vi "SSC Digital Clock Generator Initiate.vi"(0 "Digital SSC in":T1[](array[typedef]), 11 "error in":errorcluster) -> (4 "Digital SSC out":T1[](array[typedef]), 15 "error out":errorcluster)   [LabVIEW 2019]
doc: "Initiates clock generation on the device(s) connected to the specified pin(s) and pin group(s)."
uses:
  SSC Digital.ctl
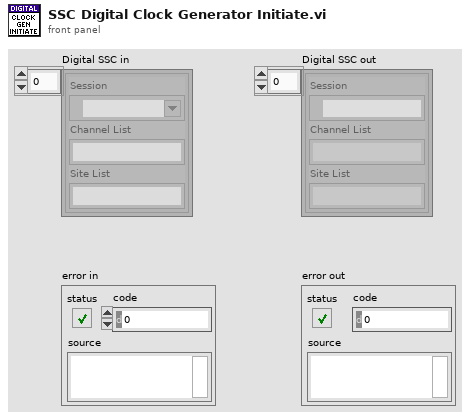
[diagram p1: front panel]
types:
  T1 = typedef "SSC Digital.ctl" = cluster{"Session":refnum<k15>, "Channel List":string, "Site List":string}
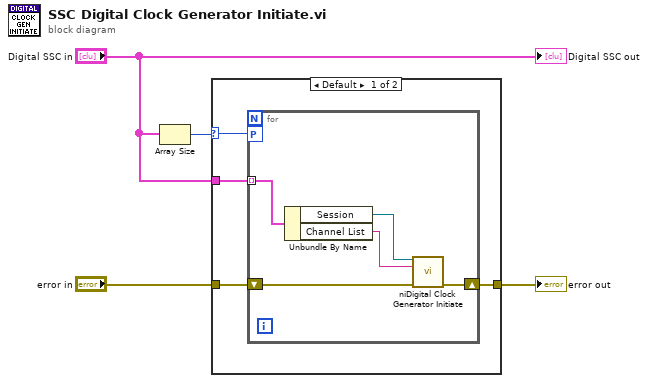
[diagram p0: block diagram]
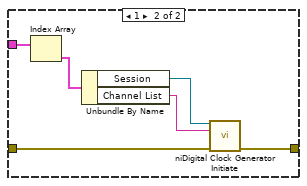
[diagram p2: hidden frame]
diagram:
  n1 = Array Size(array="Digital SSC in") -> (size(s)=w2:i32)
  n2 = case shown="Default" w2 {
    selector: w2 -> [w6 _]
    tunnel: "error in" -> [w8 w19]
    tunnel: [w7 w18] -> w3
    tunnel: "Digital SSC in" -> [w5 w17]
    frame Default {
      n3 = for {
        workers-P: w6 -> [_]
        tunnel: w5 -> [w12] mode=indexing
        shift-right: [w9] -> w7
        shift-left: w8 -> [w13]
        n4 = Unbundle By Name(w12) -> ("Session"=w11:refnum<k15>, "Channel List"=w10:string)
        n5 = call <instrlib>:"niDigital Clock Generator Initiate.vi"("instrument handle"=w11, "channel list"=w10, "error in"=w13) -> ("error out"=w9:errorcluster)  [unwired: 11 in, 1 out]
      }
    }
    frame 1 {
      n6 = Index Array(array=w17) -> (element=w14:T1)  [unwired: 1 in]
      n7 = Unbundle By Name(w14) -> ("Session"=w16:refnum<k15>, "Channel List"=w15:string)
      n8 = call <instrlib>:"niDigital Clock Generator Initiate.vi"("instrument handle"=w16, "channel list"=w15, "error in"=w19) -> ("error out"=w18:errorcluster)  [unwired: 11 in, 1 out]
    }
  }
  "error out" <- w3
  "Digital SSC out" <- "Digital SSC in"
